vi "Created.vi"(8 "Created Alias":string, 9 "Is Priority":bool, 10 "Msg":refnum<class "Msg.lvclass">, 11 "Base Actor in":refnum<class "Base Actor.lvclass">) -> (3 "Base Actor out":refnum<class "Base Actor.lvclass">)   [LabVIEW 2020, in "jettl.lvlib" / "Actor.lvlib" / "Base Actor.lvclass"]
uses:
  Base Actor.lvclass
  Error/Error.lvlib
  Sender/Relation.ctl
  Sender/Sender.lvlib
  Msg/Msg.lvclass
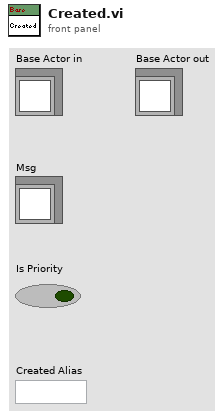
[diagram p1: front panel]
types:
  T1 = typedef "jettl.lvlib/Actor.lvlib/Implemented Msgs.ctl" = set{refnum<class "Msg.lvclass">}
  T2 = typedef "jettl.lvlib/Sender.lvlib/Relation.ctl" = enum16{"Self", "Creator", "Created"}
  T3 = typedef "jettl.lvlib/Actor.lvlib/Attributes.ctl" = cluster{"Alias":string, "Address":refnum<user-event>, "Implemented Msgs":T1, "Path":path}
  T4 = typedef "jettl.lvlib/Actor.lvlib/Alias to Created Attributes.ctl" = map{string, T3}
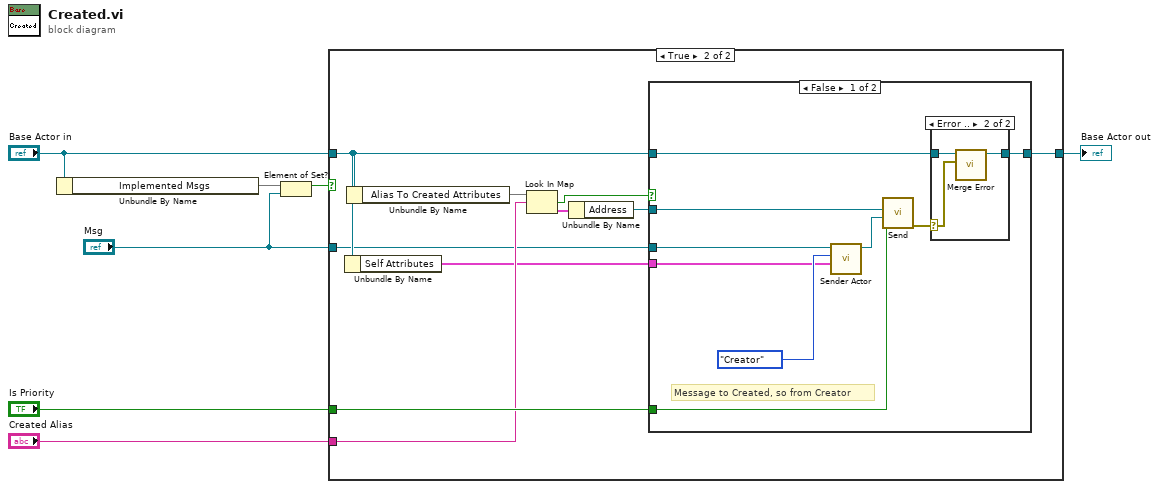
[diagram p0: block diagram]
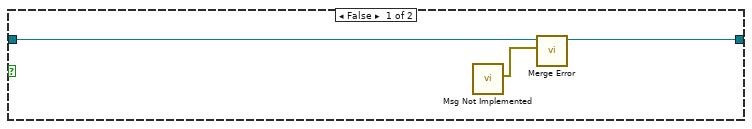
[diagram p2: hidden frame]
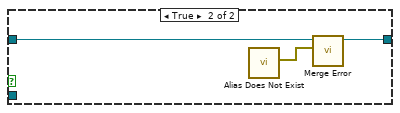
[diagram p4: hidden frame]
diagram:
  n1 = Unbundle By Name("Base Actor in") -> ("Implemented Msgs"=w3:T1)
  n2 = Element of Set?(10:"Msg", 11:w3) -> (3:w1:bool)
  n3 = case shown="True" w1 {
    tunnel: [w8 w20] -> w7
    tunnel: "Is Priority" -> [_ w19]
    tunnel: "Created Alias" -> [_ w18]
    tunnel: "Base Actor in" -> [w9 w13]
    tunnel: "Msg" -> [_ w12]
    frame False {
      n4 = call "Msg Not Implemented.vi"() -> ("Error"=w10:errorcluster)  [unwired: 11 in]
      n5 = call-dynamic "Merge Error.vi"("Error"=w10, "Base Actor in"=w9) -> ("Base Actor out"=w8:refnum<class "Base Actor.lvclass">)  [unwired: 9 in]
    }
    frame True {
      n6 = Unbundle By Name(w13) -> ("Self Attributes"=w11:T3)
      n7 = Unbundle By Name(w13) -> ("Alias To Created Attributes"=w16:T4)
      n8 = Look In Map(map=w16, key=w18) -> (key not found?=w17:bool, value=w15:T3)  [unwired: 1 in]
      n9 = Unbundle By Name(w15) -> ("Address"=w14:refnum<user-event>)
      n10 = case shown="False" w17 {
        tunnel: w13 -> [w28 w36]
        tunnel: [w27 w35] -> w20
        tunnel: w19 -> [w26 _]
        tunnel: w14 -> [w25 _]
        tunnel: w12 -> [w23 _]
        tunnel: w11 -> [w21 _]
        frame False {
          # "Message to Created, so from Creator"
          n11 = call "Sender Actor.vi"("Self Attributes"=w21, "Relation"=Relation."Creator", "Msg in"=w23) -> ("Msg out"=w24:refnum<class "Msg.lvclass">)  [unwired: 8 in]
          n12 = call "Send.vi"("Is Priority"=w26, "Msg"=w24, "Address"=w25) -> ("error out"=w29:errorcluster)  [unwired: 8 in]
          n13 = case shown="Error .." w29 {
            selector: w29 -> [_ w31]
            tunnel: [w30 w33] -> w27
            tunnel: w28 -> [w30 w32]
            frame No Error {
            }
            frame Error {
              n14 = call-dynamic "Merge Error.vi"("Error"=w31, "Base Actor in"=w32) -> ("Base Actor out"=w33:refnum<class "Base Actor.lvclass">)  [unwired: 9 in]
            }
          }
        }
        frame True {
          n15 = call "Alias Does Not Exist.vi"() -> ("Error"=w34:errorcluster)  [unwired: 11 in]
          n16 = call-dynamic "Merge Error.vi"("Error"=w34, "Base Actor in"=w36) -> ("Base Actor out"=w35:refnum<class "Base Actor.lvclass">)  [unwired: 9 in]
        }
      }
    }
  }
  "Base Actor out" <- w7
